vi "n load z table.vi"(7 "c":dbl, 8 "error in (no error)":errorcluster, 9 "b":dbl, 10 "a":dbl, 11 "n":u16) -> (0 "error out":errorcluster, 3 "function return":i16)   [LabVIEW 2015, in "SCANalone4x64.lvlib"]
doc: "__declspec(dllimport) short __stdcall n_load_z_table(unsigned short n, double a, double b, double c);"
uses:
  <userlib>/SCANalone4x64/SCANalone4x64.lvlib
  <userlib>/SCANalone4x64/SCANalone4x64.dll
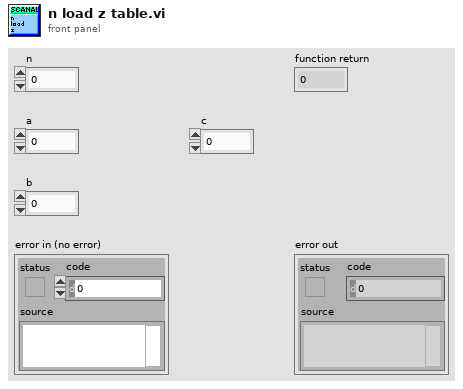
[diagram p1: front panel]
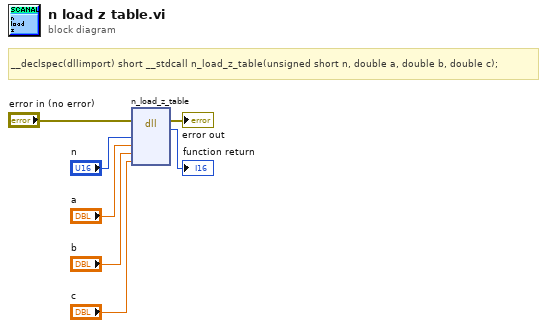
[diagram p0: block diagram]
diagram:
  # "__declspec(dllimport) short __stdcall n_load_z_table(unsigned short n, double a, double b, double c);"
  n1 = dll-call lib="C:/Program Files/National Instruments/LabVIEW 2015/user.lib/SCANalone4x64/SCANalone4x64.*" fn="n_load_z_table"(error in="error in (no error)", "n"="n", "a"="a", "b"="b", "c"="c") -> (error out=→"error out":errorcluster, →"function return":i16)  [unwired: 6 in, 1 out]
